vi "Circle Line Profile.vi"() -> ()   [LabVIEW 2020]
doc: "An example on creating circular line profiles and edge detection in images.\nThis is done in several steps in order for developers to implement custom deviations on the profile and edge detection algorthm."
uses:
  <vilib>/Natan Biesmans/G2CPU GPU and CPU HPC Toolkit/G2CPU Libraries/Arrays/1DArray/f32/1D Array f32.lvclass
  C:/Program Files/National Instruments/LabVIEW 2025/vi.lib/Natan Biesmans/G2CPU GPU and CPU HPC Toolkit/G2CPU Libraries/Arrays/Array/Array Prototype.lvclass
  <vilib>/Natan Biesmans/G2CPU GPU and CPU HPC Toolkit/G2CPU Libraries/Arrays/1DArray/s32/1D Array s32.lvclass
  <vilib>/Natan Biesmans/G2CPU GPU and CPU HPC Toolkit/G2CPU Libraries/Arrays/1DArray/binary/1D Array binary.lvclass
  <vilib>/Natan Biesmans/G2CPU GPU and CPU HPC Toolkit/G2CPU Libraries/Arrays/Array/Array Prototype.lvclass/Array Prototype.ctl
  d3694d7b-9dfe-405b-b9c4-7ff133e75b81.vi
  e057286f-6301-4877-a5f8-2699590e3ef1.vi
  4f9da12a-d444-4040-a731-8b8789de5e48.vi
  c4841cc8-a514-4b7d-9460-811ee35b1201.vi
  354f25d9-7e9d-402d-a78e-930992bf622e.vi
  423ebf9f-5cfd-4be0-9bdd-41ed530adbff.vi
  ea61818c-3b58-4232-a310-1485ca034f5f.vi
  74b37fc3-56f5-430a-b3d3-6291b5f91b15.vi
  28bd2a9c-5ab4-4101-b707-7d98e09d99f8.vi
  2434643f-ab2a-4f36-a25a-f7311a25892c.vi
  62b52a4d-f370-4dbd-b123-e838302b63d5.vi
  504b4024-6195-4238-b33a-f7e6d7e0e26f.vi
  af7bdef9-2812-4f13-ac58-5c4d8455468f.vi
  b1dfb2c7-4f4c-4c17-98fd-410d1d924a91.vi
  5a1d1dd8-1329-4c85-9c9c-9a9e781ea555.vi
  <vilib>/Natan Biesmans/G2CPU GPU and CPU HPC Toolkit/G2CPU Libraries/Arrays/SubVI/Array Sizes to Dim Cluster.vi
  d3694d7b-9dfe-405b-b9c4-7ff133e75b81.vi/3a9a0f39-20d0-42ec-98d3-19db30a3fafd.vi
  <vilib>/Natan Biesmans/G2CPU GPU and CPU HPC Toolkit/ArrayFire Driver/VIs/Run as Multi Device.vi
  <vilib>/Natan Biesmans/G2CPU GPU and CPU HPC Toolkit/G2CPU Libraries/Runtime Licensing/G2CPU License Check.vi
  e057286f-6301-4877-a5f8-2699590e3ef1.vi/3a9a0f39-20d0-42ec-98d3-19db30a3fafd.vi
  4f9da12a-d444-4040-a731-8b8789de5e48.vi/3a9a0f39-20d0-42ec-98d3-19db30a3fafd.vi
  c4841cc8-a514-4b7d-9460-811ee35b1201.vi/3a9a0f39-20d0-42ec-98d3-19db30a3fafd.vi
  354f25d9-7e9d-402d-a78e-930992bf622e.vi/3a9a0f39-20d0-42ec-98d3-19db30a3fafd.vi
  423ebf9f-5cfd-4be0-9bdd-41ed530adbff.vi/3a9a0f39-20d0-42ec-98d3-19db30a3fafd.vi
  ea61818c-3b58-4232-a310-1485ca034f5f.vi/3a9a0f39-20d0-42ec-98d3-19db30a3fafd.vi
  74b37fc3-56f5-430a-b3d3-6291b5f91b15.vi/ef94ed2d-c4e6-48dc-8bdb-249d71a97973.vi
  <vilib>/Natan Biesmans/G2CPU GPU and CPU HPC Toolkit/G2CPU Libraries/Arrays/Array/G2CPU Get Array Pointer.vi
  28bd2a9c-5ab4-4101-b707-7d98e09d99f8.vi/ef94ed2d-c4e6-48dc-8bdb-249d71a97973.vi
  2434643f-ab2a-4f36-a25a-f7311a25892c.vi/ef94ed2d-c4e6-48dc-8bdb-249d71a97973.vi
  62b52a4d-f370-4dbd-b123-e838302b63d5.vi/ef94ed2d-c4e6-48dc-8bdb-249d71a97973.vi
  504b4024-6195-4238-b33a-f7e6d7e0e26f.vi/ef94ed2d-c4e6-48dc-8bdb-249d71a97973.vi
  af7bdef9-2812-4f13-ac58-5c4d8455468f.vi/ef94ed2d-c4e6-48dc-8bdb-249d71a97973.vi
  b1dfb2c7-4f4c-4c17-98fd-410d1d924a91.vi/ef94ed2d-c4e6-48dc-8bdb-249d71a97973.vi
  5a1d1dd8-1329-4c85-9c9c-9a9e781ea555.vi/ef94ed2d-c4e6-48dc-8bdb-249d71a97973.vi
  <vilib>/Natan Biesmans/G2CPU GPU and CPU HPC Toolkit/G2CPU Libraries/Arrays/2DArray/f32/2D Array f32.lvclass
  <vilib>/Natan Biesmans/G2CPU GPU and CPU HPC Toolkit/G2CPU Libraries/Arrays/1DArray/u32/1D Array u32.lvclass
  <vilib>/Natan Biesmans/G2CPU GPU and CPU HPC Toolkit/G2CPU Libraries/File IO/Images/G2CPU Load 32b Image.vi
  <vilib>/Natan Biesmans/G2CPU GPU and CPU HPC Toolkit/G2CPU Libraries/Arrays/Array/G2CPU Get Data Type.vi
  <vilib>/Natan Biesmans/G2CPU GPU and CPU HPC Toolkit/G2CPU Libraries/Arrays/Array/G2CPU Array Element Count.vi
  <vilib>/Natan Biesmans/G2CPU GPU and CPU HPC Toolkit/ArrayFire Driver/VIs/is scalar.vi
  <vilib>/Natan Biesmans/G2CPU GPU and CPU HPC Toolkit/ArrayFire Driver/VIs/is empty.vi
  <vilib>/Natan Biesmans/G2CPU GPU and CPU HPC Toolkit/ArrayFire Driver/subvi/Error Converter (ErrCode or Status).vi
  <vilib>/Natan Biesmans/G2CPU GPU and CPU HPC Toolkit/G2CPU Libraries/Arrays/SubVI/G2CPU State.vi
  <vilib>/NI License Manager/Open Session.vi
  <vilib>/NI License Manager/Check License Status.vi
  <vilib>/NI License Manager/Check License Status (Single).vi
  <vilib>/NI License Manager/Activate License.vi
  <vilib>/NI License Manager/Activate License (Single).vi
  <vilib>/NI License Manager/Close Session.vi
  <vilib>/Natan Biesmans/G2CPU GPU and CPU HPC Toolkit/G2CPU Libraries/Arrays/Array/G2CPU Set Array Pointer.vi
  <vilib>/Natan Biesmans/G2CPU GPU and CPU HPC Toolkit/G2CPU Libraries/Arrays/DataTypes/f32/f32.lvclass
  <vilib>/Natan Biesmans/G2CPU GPU and CPU HPC Toolkit/G2CPU Libraries/Arrays/2DArray/2D Array Prototype.lvclass
  <vilib>/Natan Biesmans/G2CPU GPU and CPU HPC Toolkit/G2CPU Libraries/Arrays/1DArray/1D Array Prototype.lvclass
  <vilib>/Natan Biesmans/G2CPU GPU and CPU HPC Toolkit/G2CPU Libraries/File IO/G2CPU File IO.lvlib
  G2CPU Line Profile.lvlib
  <vilib>/Natan Biesmans/G2CPU GPU and CPU HPC Toolkit/G2CPU Libraries/Arrays/Array/Array Prototype.lvclass
panel:
  in  "Rising Edge":bool[](array[boolean])=[TRUE, FALSE]
  in  "Amounts of Lines":i32[](array[numeric])=[8, 20]
  in  "Treshold":i32[](array[numeric])=[50, 50]
  in  "Outer Radius":sgl[](array[numeric])=[100.0, 150.0] format="%#_g px"
  in  "Inner Radius":sgl[](array[numeric])=[10.0, 10.0] format="%#_g px"
  in  "Center Y":sgl[](array[numeric])=[160.0, 160.0] format="%#_g px"
  in  "Center X":sgl[](array[numeric])=[160.0, 160.0] format="%#_g px"
  in  "Image File":path=path "C:/Program Files/ArrayFire/v3/examples/images/donut.png"
  out "Original Image":sgl[][](graph)
  out "Line Profiles":sgl[][](graph)
  # "Circle Location"
  # "Circle Sizing"
  # "Edge Detection Parameters"
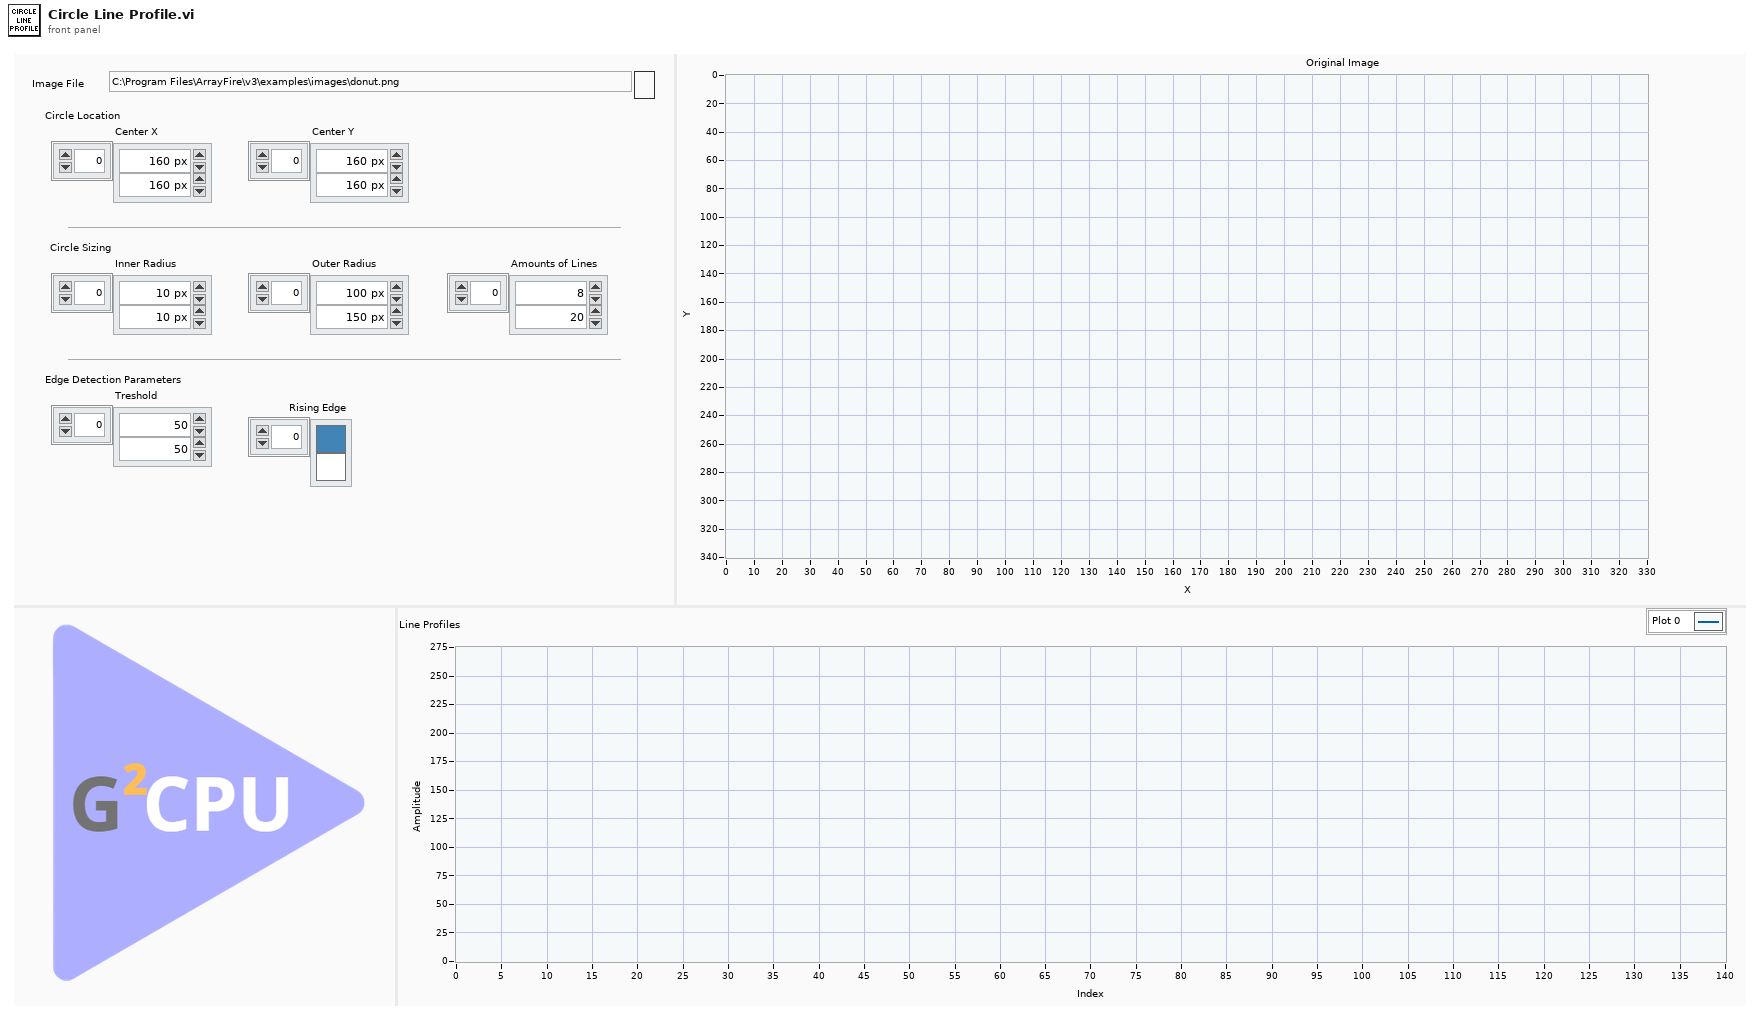
[diagram p1: front panel]
types:
  T1 = cluster{"Rising Edge?":refnum<class "1D Array binary.lvclass">, "Treshold":refnum<class "1D Array s32.lvclass">}
  T2 = cluster{"Center X":refnum<class "1D Array f32.lvclass">, "Center Y":refnum<class "1D Array f32.lvclass">, "Inner Radius":refnum<class "1D Array f32.lvclass">, "Outer Radius":refnum<class "1D Array f32.lvclass">, "Amounts of Lines":refnum<class "1D Array s32.lvclass">}
  T3 = cluster{"Auto Release Line Indexers (Enabled)":bool, "Auto Release Keys (Enabled)":bool}
  T4 = cluster{"Points 1 X":refnum<class "1D Array f32.lvclass">, "Points 1 Y":refnum<class "1D Array f32.lvclass">, "Points 2 X":refnum<class "1D Array f32.lvclass">, "Points 2 Y":refnum<class "1D Array f32.lvclass">, "Keys":refnum<class "1D Array u32.lvclass">}
  T5 = cluster{"Line Indexes":refnum<class "2D Array f32.lvclass">, "Keys":refnum<class "2D Array u32.lvclass">, "Index Overflow":u64}
  T6 = cluster{"Line Profiles":refnum<class "2D Array f32.lvclass">, "Keys":refnum<class "2D Array u32.lvclass">}
  T7 = cluster{"X Coordinates":refnum<class "1D Array f32.lvclass">, "Y Coordinates":refnum<class "1D Array f32.lvclass">, "Keys":refnum<class "1D Array u32.lvclass">}
  T8 = cluster{"Name":string, "Color":u32, "Style":u8, "Point Style":u8, "Name Visible":bool, "Allow Drag":bool, "Annotation Mode":u32, "Plot":i32, "Index":i32, "Position":cluster{"X":dbl, "Y":dbl}, "X Scale":u32, "Y Scale":u32, "Show Arrow":bool, "Lock Name":bool, "Plot Area":i32, "Label Offset":cluster{"X":dbl, "Y":dbl}}
  T9 = cluster{"Name":string, "Color":u32, "Style":u8, "Point Style":u8, "Name Visible":bool, "Allow Drag":bool, "Annotation Mode":u32, "Plot":i32, "Index":i32, "Position":cluster{"X":dbl, "Y":dbl}, "X Scale":u32, "Y Scale":u32, "Show Arrow":bool, "Lock Name":bool, "Plot Area":i32, "Label Offset":cluster{"X":dbl, "Y":dbl}}[]
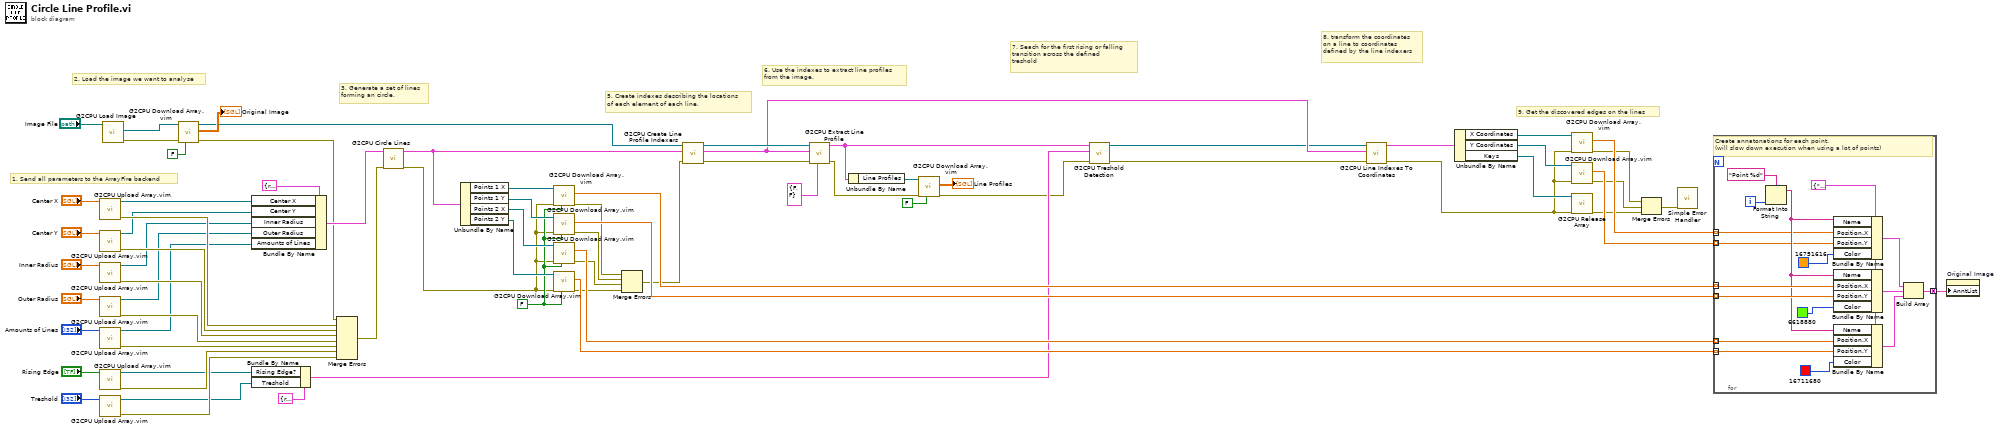
[diagram p0: block diagram]
diagram:
  w46 = FALSE ("Auto Release Array In")
  # "9. Get the discovered edges on the lines"
  # "8. transform the coordinates\non a line to coordinates\ndefined by the line indexers"
  # "7. Seach for the first rising or falling\ntransition across the defined \ntreshold"
  # "6. Use the indexes to extract line profiles \nfrom the image."
  # "5. Create indexes describing the locations\nof each element of each line."
  # "3. Generate a set of lines \nforming an circle."
  # "2. Load the image we want to analyse"
  # "1. Send all parameters to the ArrayFire backend"
  n1 = call "G2CPU Upload Array.vim"("Data"="Center X") -> ("error out"=w73:errorcluster, "Array"=w52:refnum<class "1D Array f32.lvclass">)  [unwired: 9 in]
  n2 = call "G2CPU Upload Array.vim"("Data"="Center Y") -> ("error out"=w72:errorcluster, "Array"=w53:refnum<class "1D Array f32.lvclass">)  [unwired: 9 in]
  n3 = call "G2CPU Upload Array.vim"("Data"="Inner Radius") -> ("error out"=w71:errorcluster, "Array"=w54:refnum<class "1D Array f32.lvclass">)  [unwired: 9 in]
  n4 = call "G2CPU Upload Array.vim"("Data"="Outer Radius") -> ("error out"=w70:errorcluster, "Array"=w55:refnum<class "1D Array f32.lvclass">)  [unwired: 9 in]
  n5 = call "G2CPU Upload Array.vim"("Data"="Amounts of Lines") -> ("error out"=w69:errorcluster, "Array"=w56:refnum<class "1D Array s32.lvclass">)  [unwired: 9 in]
  n6 = call "G2CPU Upload Array.vim"("Data"="Rising Edge") -> ("error out"=w68:errorcluster, "Array"=w32:refnum<class "1D Array binary.lvclass">)  [unwired: 9 in]
  n7 = call "G2CPU Upload Array.vim"("Data"="Treshold") -> ("error out"=w67:errorcluster, "Array"=w31:refnum<class "1D Array s32.lvclass">)  [unwired: 9 in]
  n8 = call-poly <vilib>:"G2CPU Load Image.vi"("Filename"="Image File") -> ("error out"=w65:errorcluster, "Array out"=w66:refnum<class "2D Array f32.lvclass">)  [unwired: 7 in, 2 out]
  n9 = call "G2CPU Download Array.vim"("Auto Release Array In"=FALSE, "error in (no error)"=w65, "Array in"=w66) -> ("error out"=w25:errorcluster, "Array Data"=→"Original Image":sgl[][], "Array Out"=w40:refnum<class "2D Array f32.lvclass">)  [unwired: 6 in]
  n10 = Bundle By Name(cluster=T2 {"Center X"=refnum, "Center Y"=refnum, "Inner Radius"=refnum, "Outer Radius"=refnum, "Amounts of Lines"=refnum} ("Circles Parameters"), "Center X"=w52, "Center Y"=w53, "Inner Radius"=w54, "Outer Radius"=w55, "Amounts of Lines"=w56) -> (w57:T2)
  n11 = Bundle By Name(cluster=T1 {"Rising Edge?"=refnum, "Treshold"=refnum} ("Treshold Parameters"), "Rising Edge?"=w32, "Treshold"=w31) -> (w33:T1)
  n12 = Merge Errors(w25, w73, w72, w71, w70, w69, w68, w67) -> (w24:errorcluster)
  n13 = call "G2CPU Circle Lines.vi"("error in (no error)"=w24, "Circles Parameters"=w57) -> ("error out"=w13:errorcluster, "Lines"=w51:T4)  [unwired: 8 in]
  n14 = Unbundle By Name(w51) -> ("Points 1 X"=w47:refnum<class "1D Array f32.lvclass">, "Points 1 Y"=w48:refnum<class "1D Array f32.lvclass">, "Points 2 X"=w49:refnum<class "1D Array f32.lvclass">, "Points 2 Y"=w50:refnum<class "1D Array f32.lvclass">)
  n15 = call "G2CPU Download Array.vim"("Auto Release Array In"=w46, "error in (no error)"=w13, "Array in"=w47) -> ("error out"=w17:errorcluster, "Array Data"=w44:sgl[])  [unwired: 6 in, 1 out]
  n16 = call "G2CPU Download Array.vim"("Auto Release Array In"=w46, "error in (no error)"=w13, "Array in"=w48) -> ("error out"=w16:errorcluster, "Array Data"=w43:sgl[])  [unwired: 6 in, 1 out]
  n17 = call "G2CPU Download Array.vim"("Auto Release Array In"=w46, "error in (no error)"=w13, "Array in"=w49) -> ("error out"=w15:errorcluster, "Array Data"=w42:sgl[])  [unwired: 6 in, 1 out]
  n18 = call "G2CPU Download Array.vim"("Auto Release Array In"=w46, "error in (no error)"=w13, "Array in"=w50) -> ("error out"=w14:errorcluster, "Array Data"=w41:sgl[])  [unwired: 6 in, 1 out]
  n19 = Merge Errors(w17, w16, w15, w14) -> (w12:errorcluster)
  n20 = call "G2CPU Create Line Profile Indexers.vi"("error in (no error)"=w12, "Lines"=w51, "Greyscale Image In"=w40) -> ("error out"=w60:errorcluster, "Line Indexers"=w61:T5, "Greyscale Image Out (inplace)"=w62:refnum<class "2D Array f32.lvclass">)  [unwired: 6 in]
  n21 = call "G2CPU Extract Line Profile.vi"("Auto Release Line Indexers"=T3 {"Auto Release Line Indexers (Enabled)"=FALSE, "Auto Release Keys (Enabled)"=FALSE}, "error in (no error)"=w60, "Line Indexers"=w61, "Greyscale Image In"=w62) -> ("error out"=w11:errorcluster, "Line Profiles Out"=w36:T6)  [unwired: 6 in]
  n22 = Unbundle By Name(w36) -> ("Line Profiles"=w37:refnum<class "2D Array f32.lvclass">)
  n23 = call "G2CPU Download Array.vim"("Auto Release Array In"=FALSE, "error in (no error)"=w11, "Array in"=w37) -> ("error out"=w10:errorcluster, "Array Data"=→"Line Profiles":sgl[][])  [unwired: 6 in, 1 out]
  n24 = call "G2CPU Treshold Detection.vi"("error in (no error)"=w10, "Treshold Parameters"=w33, "Line Profiles"=w36) -> ("error out"=w38:errorcluster, "Edge Indexes out"=w39:refnum<class "1D Array f32.lvclass">)  [unwired: 7 in]
  n25 = call "G2CPU Line Indexes To Coordinates.vi"("error in (no error)"=w38, "Line Indexers"=w61, "Point of Interest on Lines"=w39) -> ("error out"=w22:errorcluster, "Coordinates Out"=w35:T7)  [unwired: 7 in]
  n26 = Unbundle By Name(w35) -> ("X Coordinates"=w27:refnum<class "1D Array f32.lvclass">, "Y Coordinates"=w28:refnum<class "1D Array f32.lvclass">, "Keys"=w26:refnum<class "1D Array u32.lvclass">)
  n27 = call "G2CPU Download Array.vim"("error in (no error)"=w22, "Array in"=w27) -> ("error out"=w21:errorcluster, "Array Data"=w30:sgl[])  [unwired: 7 in, 1 out]
  n28 = call "G2CPU Download Array.vim"("error in (no error)"=w22, "Array in"=w28) -> ("error out"=w19:errorcluster, "Array Data"=w29:sgl[])  [unwired: 7 in, 1 out]
  n29 = call <vilib>:"G2CPU Release Array.vi"("error in (no error)"=w22, "Array in"=w26) -> ("error out"=w18:errorcluster)  [unwired: 9 in]
  n30 = Merge Errors(w21, w19, w18) -> (w20:errorcluster)
  n31 = call <vilib>:"Simple Error Handler.vi"("error in (no error)"=w20) -> ()  [unwired: 4 in, 5 out]
  n32 = for {
    tunnel: [w86] -> w45 mode=concatenating
    tunnel: w44 -> [w83] mode=indexing
    tunnel: w43 -> [w82] mode=indexing
    tunnel: w42 -> [w81] mode=indexing
    tunnel: w41 -> [w80] mode=indexing
    tunnel: w30 -> [w76] mode=indexing
    tunnel: w29 -> [w75] mode=indexing
    i -> [w85]
    w78 = T8 {"Name"="azerty", "Color"=16776960, "Style"=4, "Point Style"=13, "Name Visible"=FALSE, "Allow Drag"=FALSE, "Annotation Mode"=0, "Plot"=-1, "Index"=0, "Position"={"X"=162.8968713789108, "Y"=222.19554030874787}, "X Scale"=0, "Y Scale"=0, "Show Arrow"=FALSE, "Lock Name"=FALSE, "Plot Area"=0, "Label Offset"={"X"=0.0, "Y"=-11.663807890222984}}
    # "Create annatonations for each point.\n(will slow down execution when using a lot of points)"
    n33 = Format Into String(format string="Point %d", w85) -> (resulting string=w77:string)  [unwired: 2 in, 1 out]
    n34 = Bundle By Name(cluster=w78, "Name"=w77, "Position.X"=w76, "Position.Y"=w75, "Color"=u32 16751616) -> (w74:T8)
    n35 = Bundle By Name(cluster=w78, "Name"=w77, "Position.X"=w83, "Position.Y"=w82, "Color"=u32 6618880) -> (w87:T8)
    n36 = Bundle By Name(cluster=w78, "Name"=w77, "Position.X"=w81, "Position.Y"=w80, "Color"=u32 16711680) -> (w88:T8)
    n37 = Build Array(w74, w87, w88) -> (w86:T9)
  }
  n38 = property on="Original Image" class="IntGraph (strict)"("AnntList"=w45) -> ()  [unwired: 2 in, 2 out]
